vi "Apply_0V_to_J5000-1.vi"(3 "error in":errorcluster) -> (10 "error out":errorcluster)   [LabVIEW 2015]
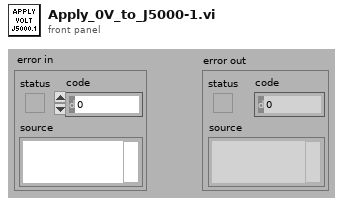
[diagram p1: front panel]
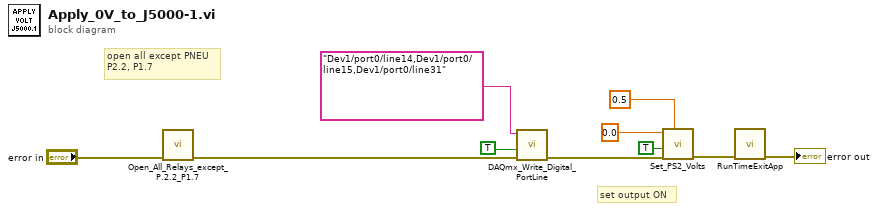
[diagram p0: block diagram]
diagram:
  # "set output ON"
  # "open all except PNEU\nP2.2, P1.7"
  n1 = call "Open_All_Relays_except_P.2.2_P1.7.vi"("error in"="error in") -> ("error out"=w2:errorcluster)  [unwired: 8 in]
  n2 = call "DAQmx_Write_Digital_PortLine.vi"("Device/Ports/Lines"="Dev1/port0/line14,Dev1/port0/line15,Dev1/port0/line31", "Boolean"=TRUE, "error in"=w2) -> ("error out"=w8:errorcluster)  [unwired: 6 in, 1 out]
  n3 = call "Set_PS2_Volts.vi"("delay (secs)"=0.5, "error in"=w8, "Output on/off"=TRUE, "Output Voltage"=0.0 ("Output Voltage (0)")) -> ("error out"=w7:errorcluster)  [unwired: 5 in, 2 out]
  n4 = call "RunTimeExitApp.vi"("error in (no error)"=w7) -> ("error out"=→"error out":errorcluster)  [unwired: 10 in]
